vi "Load File.vi"(6 "replace if found? (F)":bool, 8 "error in (no error)":errorcluster, 9 "create file if necessary? (T)":bool=TRUE, 10 "configuration file path":path, 11 "Configuration Session in":refnum<class "Configuration Session.lvclass">) -> (0 "error out":errorcluster, 1 "file created?":bool, 3 "Configuration Session out":refnum<class "Configuration Session.lvclass">, 4 "file replaced?":bool)   [LabVIEW 2017, in "DSF Configuration.lvlib" / "Configuration Session.lvclass"]
uses:
  Configuration Session.lvclass
  Configuration Session.lvclass/Configuration Session.ctl
  DSF Configuration API/Private/Controls/Session/DSF Config Data.ctl
  DSF Configuration API/Private/Controls/DSF File Format/Internal.DSF Configuration.ctl
  DSF Configuration API/Public/Controls/DSF Version Info.ctl
  DSF Configuration API/Private/Controls/DSF File Format/Internal.DSF Plugin with ID.ctl
  DSF Configuration API/Private/Controls/DSF File Format/Internal.DSF Plugin Info.ctl
  DSF Configuration API/Public/Controls/DSF Timing Info.ctl
  DSF Configuration API/Private/Controls/DSF File Format/Internal.DSF Group with ID.ctl
  DSF Configuration API/Private/Controls/DSF File Format/Internal.DSF Group Info.ctl
  DSF Configuration API/Private/Controls/DSF File Format/Internal.DSF Transfer with ID.ctl
  DSF Configuration API/Private/Controls/DSF File Format/Internal.DSF Transfer Info.ctl
  DSF Configuration API/Private/Controls/DSF File Format/Internal.DSF Channel with ID.ctl
  DSF Configuration API/Private/Controls/DSF File Format/Internal.DSF Channel Info.ctl
  DSF Configuration API/Private/Controls/DSF File Format/Internal.DSF Settings with ID.ctl
  DSF Configuration API/Private/Controls/DSF File Format/Internal.DSF Settings Info.ctl
  DSF Configuration.lvlib
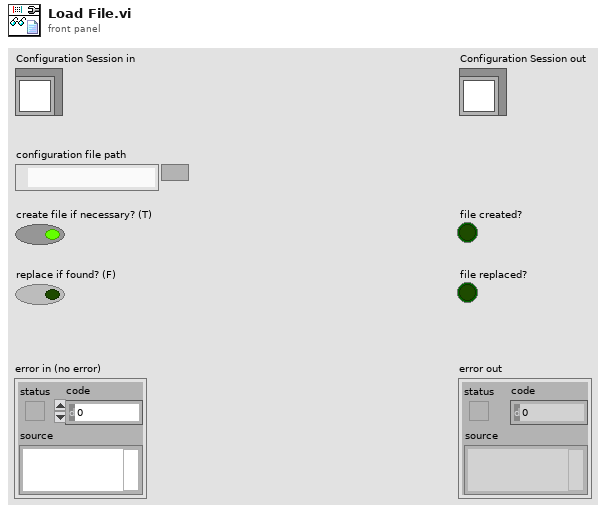
[diagram p1: front panel]
types:
  T1 = typedef "DSF Configuration.lvlib/Configuration Session.lvclass/DSF Config Data.ctl" = cluster{"dsf configuration":T2, "path":path, "dirty":bool}
  T2 = typedef "DSF Configuration.lvlib/Configuration Session.lvclass/Internal.DSF Configuration.ctl" = cluster{"dsfversion":T3, "version":T3, "plugins":T4[], "groups":T7[], "transfers":T9[], "channels":T11[], "settings":T13[]}
  T3 = typedef "DSF Configuration.lvlib/DSF Version Info.ctl" = cluster{"major":u32, "minor":u32, "fix":u32, "build":string}
  T4 = typedef "DSF Configuration.lvlib/Configuration Session.lvclass/Internal.DSF Plugin with ID.ctl" = cluster{"id":string, "values":T5}
  T5 = typedef "DSF Configuration.lvlib/Configuration Session.lvclass/Internal.DSF Plugin Info.ctl" = cluster{"type":string, "timing":T6, "group ids":string[], "settings id":string}
  T6 = typedef "DSF Configuration.lvlib/DSF Timing Info.ctl" = cluster{"priority":u64, "decimation":u64, "offset":u64}
  T7 = typedef "DSF Configuration.lvlib/Configuration Session.lvclass/Internal.DSF Group with ID.ctl" = cluster{"id":string, "values":T8}
  T8 = typedef "DSF Configuration.lvlib/Configuration Session.lvclass/Internal.DSF Group Info.ctl" = cluster{"direction":i32, "timing":T6, "transfer ids":string[], "settings id":string}
  T9 = typedef "DSF Configuration.lvlib/Configuration Session.lvclass/Internal.DSF Transfer with ID.ctl" = cluster{"id":string, "values":T10}
  T10 = typedef "DSF Configuration.lvlib/Configuration Session.lvclass/Internal.DSF Transfer Info.ctl" = cluster{"byte order":i32, "channel ids":string[], "settings id":string}
  T11 = typedef "DSF Configuration.lvlib/Configuration Session.lvclass/Internal.DSF Channel with ID.ctl" = cluster{"id":string, "values":T12}
  T12 = typedef "DSF Configuration.lvlib/Configuration Session.lvclass/Internal.DSF Channel Info.ctl" = cluster{"count":u64, "buffer offset":u64, "data type":i32, "settings id":string}
  T13 = typedef "DSF Configuration.lvlib/Configuration Session.lvclass/Internal.DSF Settings with ID.ctl" = cluster{"id":string, "values":T14}
  T14 = typedef "DSF Configuration.lvlib/Configuration Session.lvclass/Internal.DSF Settings Info.ctl" = cluster{"key":string, "value":string}[]
  T15 = enum16{"open", "replace", "create", "open or create", "replace or create", "replace or create with confirmation"}
  T16 = typedef "DSF Configuration.lvlib/Configuration Session.lvclass/Config Data Ref.ctl" = refnum<data-value>
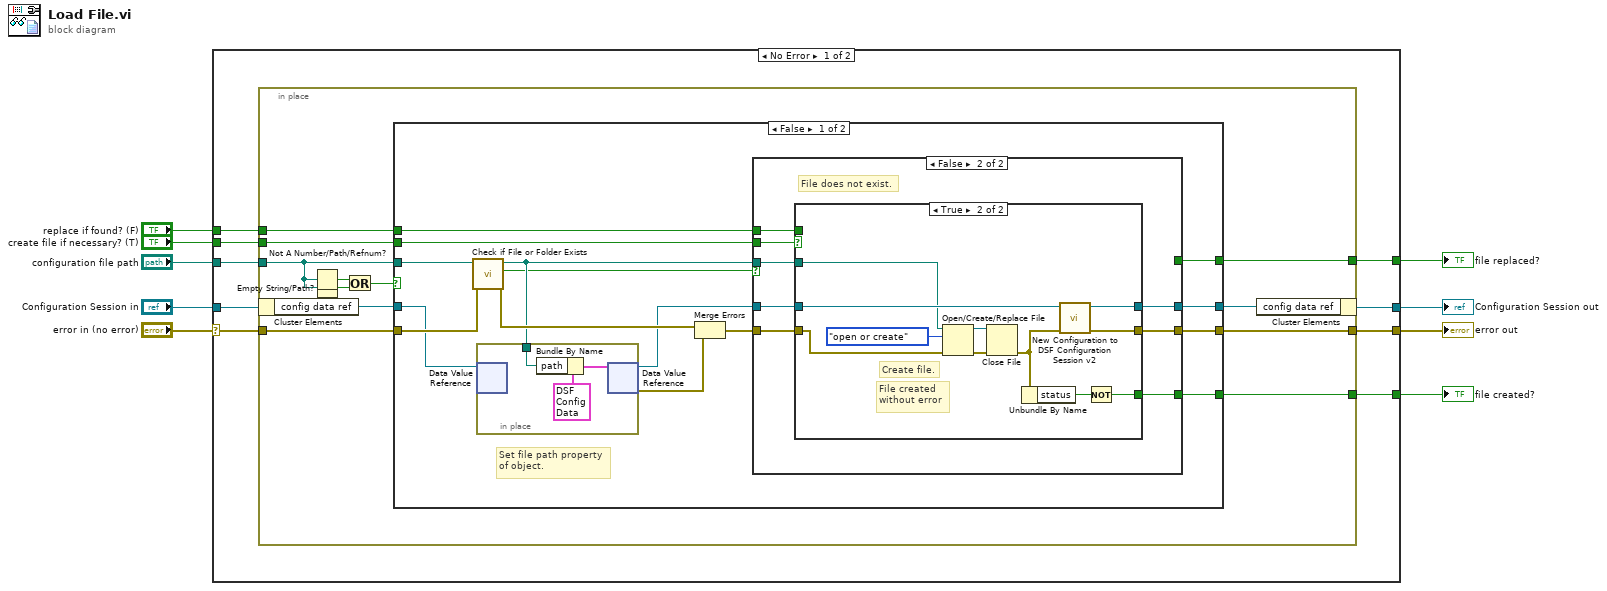
[diagram p0: block diagram]
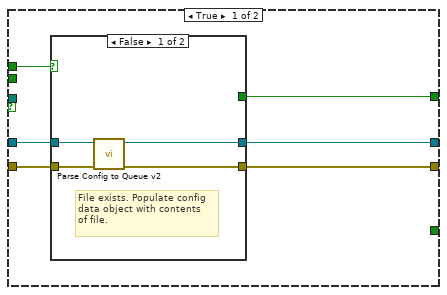
[diagram p2: hidden frame]
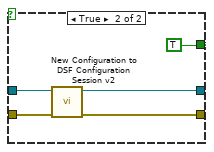
[diagram p3: hidden frame]
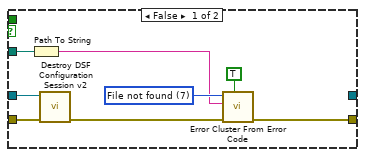
[diagram p4: hidden frame]
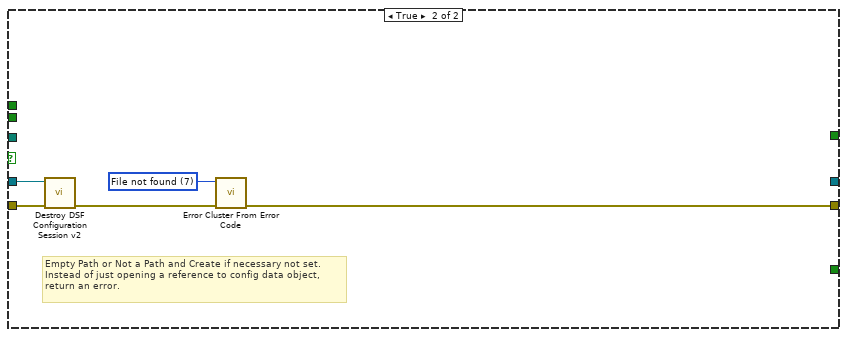
[diagram p5: hidden frame]
diagram:
  n1 = case shown="No Error" "error in (no error)" {
    selector: "error in (no error)" -> [w10 w96]
    tunnel: [w18 w96] -> w9
    tunnel: "Configuration Session in" -> [w17 w97]
    tunnel: "replace if found? (F)" -> [w16 _]
    tunnel: "create file if necessary? (T)" -> [w15 _]
    tunnel: [w14 w97] -> w5
    tunnel: "configuration file path" -> [w13 _]
    tunnel: [w12 _] -> w3
    tunnel: [w11 _] -> w2
    frame No Error {
      n2 = in-place {
        in-place-border: w10 -> [w30]
        in-place-border: [w29] -> w18
        in-place-border: w16 -> [w26]
        in-place-border: w15 -> [w25]
        in-place-border: w13 -> [w19]
        in-place-border: [w24] -> w12
        in-place-border: [w23] -> w11
        n3 = in-place-cluster #1(w17) -> ("config data ref"=w28:T16)
        n4 = Not A Number/Path/Refnum? ("Not A Number/Path/dsf refnum?")(number/path/refnum=w19) -> (NaN/Path/Refnum?=w21:bool)
        n5 = Empty String/Path?(string/path=w19) -> (empty?=w22:bool)
        n6 = Or(x=w21, y=w22) -> (x .or. y?=w20:bool)
        n7 = case shown="False" w20 {
          tunnel: [w45 w95] -> w29
          tunnel: w19 -> [w41 _]
          tunnel: w25 -> [w44 _]
          tunnel: w30 -> [w35 w93]
          tunnel: [w43 _] -> w27
          tunnel: [w42 _] -> w23
          tunnel: w28 -> [w31 w91]
          tunnel: w26 -> [w38 _]
          tunnel: [w37 _] -> w24
          frame False {
            # "Set file path property\nof object."
            n8 = call <vilib>:"Check if File or Folder Exists.vi"("error in (no error)"=w35, "path"=w41) -> ("error out"=w40:errorcluster, "file or folder exists?"=w32:bool, "dup path"=w36:path)  [unwired: 7 out]
            n9 = in-place {
              in-place-border: w36 -> [w48]
              n10 = in-place-dvr #2(w31) -> ()  [unwired: 2 out]
              n11 = Bundle By Name(cluster=T1 {"dsf configuration"={"dsfversion"={"major"=0, "minor"=0, "fix"=0, "build"=""}, "version"={"major"=0, "minor"=0, "fix"=0, "build"=""}, "plugins"=[], "groups"=[], "transfers"=[], "channels"=[], "settings"=[]}, "path"=path "", "dirty"=FALSE} ("config data"), "path"=w48) -> (w47:T1)
              n12 = in-place-dvr #2(w47) -> (w33:T16, w39:errorcluster)
            }
            n13 = Merge Errors(w40, w39) -> (w34:errorcluster)
            n14 = case shown="False" w32 {
              tunnel: [w53 w70] -> w45
              tunnel: w36 -> [_ w71]
              tunnel: w44 -> [_ w69]
              tunnel: w33 -> [w54 w66]
              tunnel: [w52 w67] -> w43
              tunnel: [_ w68] -> w42
              tunnel: w38 -> [w51 w65]
              tunnel: [w50 _] -> w37
              tunnel: w34 -> [w49 w64]
              frame True {
                n15 = case shown="False" w51 {
                  tunnel: w54 -> [w58 w59]
                  tunnel: [w55 w60] -> w53
                  tunnel: [w57 w62] -> w52
                  tunnel: w49 -> [w56 w61]
                  tunnel: [_ TRUE] -> w50
                  frame False {
                    # "File exists. Populate config\ndata object with contents\nof file."
                    n16 = call "Parse Config to Queue v2.vi"("error in"=w56, "config data ref in"=w58) -> ("error out"=w55:errorcluster, "config data ref out"=w57:T16)  [unwired: 8 in]
                  }
                  frame True {
                    n17 = call "New Configuration to DSF Configuration Session v2.vi"("error in"=w61, "config data ref in"=w59) -> ("error out"=w60:errorcluster, "config data ref out"=w62:T16)  [unwired: 8 in]
                  }
                }
              }
              frame False {
                # "File does not exist."
                n18 = case shown="True" w69 {
                  tunnel: w71 -> [w76 w81]
                  tunnel: [w78 w82] -> w70
                  tunnel: [_ w86] -> w68
                  tunnel: [_ w84] -> w67
                  tunnel: w66 -> [w74 w83]
                  tunnel: w65 -> [_ _]
                  tunnel: w64 -> [w72 w80]
                  frame False {
                    w79 = u16 7 items=["No error", "Argument error", "Memory is full", "Out of zone", "End of file", "File already open", "Generic file I/O error", "File not found", "File permission error", "Disk is full", "Duplicate path", "Too many files open", "System feature not enabled", "Resource file not found", "Cannot add resource", "Resource not found", "Image not found", "Image memory error", "Pen does not exist", "Config type invalid", "Config token not found", "Config parse error", "Config memory error", "Bad external code format", "Bad external code offset", "External code not present", "Null window", "Destroy window error", "Null menu", "Print aborted", "Bad print record", "Print driver error", "Windows error during printing", "Memory error during printing", "Print dialog error", "Generic print error", "Invalid device refnum", "Device not found", "Device parameter error", "Device unit error", "Cannot open device", "Device call aborted", "Generic error", "Cancelled by user", "Object ID too low", "Object ID too high", "Object not in heap", "Unknown heap", "Unknown object (invalid DefProc)", "Unknown object (DefProc not in table)", "Message out of range", "Invalid (null) method", "Unknown message", "Manager call not supported", "Bad address", "Network operation in progress", "Network operation timed out", "Connection is busy", "Network attribute not supported", "Network error", "Address in use", "System out of memory", "Connection aborted", "Connection refused", "Not connected", "Already connected", "Connection closed", "Initialization error (interapplication manager)", "Bad occurrence", "Wait on unbound occurrence handler", "Occurrence queue overflow", "Datalog type conflict", "Unused", "Unrecognized type (interapplication manager)", "Memory corrupt", "Failed to make temporary DLL", "Old CIN version", "Drag socket not found", "Failed to load drop-object", "Failed to register OLE object", "Failed to release OLE object", "Format specifier type mismatch", "Unknown format specifier", "Too few format specifiers", "Too many format specifiers", "Scan failed", "Newer CIN version", "OLE Convert", "Runtime menu error", "Password tampered", "Unknown error code"]
                    n19 = Path To String(path=w76) -> (string=w75:string)
                    n20 = call "Destroy DSF Configuration Session v2.vi"("error in (no error)"=w72, "config data ref"=w74) -> ("error out"=w73:errorcluster)  [unwired: 9 in]
                    n21 = call <vilib>:"Error Cluster From Error Code.vi"("show call chain? (False)"=TRUE, "error in (no error)"=w73, "error message (\"\")"=w75, "error code (0)"=w79) -> ("error out"=w78:errorcluster)  [unwired: 5 out]
                  }
                  frame True {
                    # "File created\nwithout error"
                    # "Create file."
                    n22 = Open/Create/Replace File(file path (use dialog)=w81, error in=w80, operation (0:open)=T15."open or create") -> (refnum out=w89:refnum<file>, error out=w90:errorcluster)  [unwired: 4 out]
                    n23 = Close File(refnum=w89, error in=w90) -> (error out=w87:errorcluster)  [unwired: 1 out]
                    n24 = Unbundle By Name(w87) -> ("status"=w88:bool)
                    n25 = call "New Configuration to DSF Configuration Session v2.vi"("error in"=w87, "config data ref in"=w83) -> ("error out"=w82:errorcluster, "config data ref out"=w84:T16)  [unwired: 8 in]
                    n26 = Not(x=w88) -> (.not. x?=w86:bool)
                  }
                }
              }
            }
          }
          frame True {
            w94 = u16 7 items=["No error", "Argument error", "Memory is full", "Out of zone", "End of file", "File already open", "Generic file I/O error", "File not found", "File permission error", "Disk is full", "Duplicate path", "Too many files open", "System feature not enabled", "Resource file not found", "Cannot add resource", "Resource not found", "Image not found", "Image memory error", "Pen does not exist", "Config type invalid", "Config token not found", "Config parse error", "Config memory error", "Bad external code format", "Bad external code offset", "External code not present", "Null window", "Destroy window error", "Null menu", "Print aborted", "Bad print record", "Print driver error", "Windows error during printing", "Memory error during printing", "Print dialog error", "Generic print error", "Invalid device refnum", "Device not found", "Device parameter error", "Device unit error", "Cannot open device", "Device call aborted", "Generic error", "Cancelled by user", "Object ID too low", "Object ID too high", "Object not in heap", "Unknown heap", "Unknown object (invalid DefProc)", "Unknown object (DefProc not in table)", "Message out of range", "Invalid (null) method", "Unknown message", "Manager call not supported", "Bad address", "Network operation in progress", "Network operation timed out", "Connection is busy", "Network attribute not supported", "Network error", "Address in use", "System out of memory", "Connection aborted", "Connection refused", "Not connected", "Already connected", "Connection closed", "Initialization error (interapplication manager)", "Bad occurrence", "Wait on unbound occurrence handler", "Occurrence queue overflow", "Datalog type conflict", "Unused", "Unrecognized type (interapplication manager)", "Memory corrupt", "Failed to make temporary DLL", "Old CIN version", "Drag socket not found", "Failed to load drop-object", "Failed to register OLE object", "Failed to release OLE object", "Format specifier type mismatch", "Unknown format specifier", "Too few format specifiers", "Too many format specifiers", "Scan failed", "Newer CIN version", "OLE Convert", "Runtime menu error", "Password tampered", "Unknown error code"]
            # "Empty Path or Not a Path and Create if necessary not set.\nInstead of just opening a reference to config data object,\nreturn an error."
            n27 = call "Destroy DSF Configuration Session v2.vi"("error in (no error)"=w93, "config data ref"=w91) -> ("error out"=w92:errorcluster)  [unwired: 9 in]
            n28 = call <vilib>:"Error Cluster From Error Code.vi"("error in (no error)"=w92, "error code (0)"=w94) -> ("error out"=w95:errorcluster)  [unwired: 1 in, 6 out]
          }
        }
        n29 = in-place-cluster #1("config data ref"=w27) -> (w14:refnum<class "Configuration Session.lvclass">)
      }
    }
    frame Error {
    }
  }
  "error out" <- w9
  "Configuration Session out" <- w5
  "file created?" <- w2
  "file replaced?" <- w3
